vi "S_param_from_frame.VI"(2 "Ref Impedance":u16=75, 3 "S-parameter Array":cdb[][](array[numeric]) format="%.2f", 4 "Frequencies (Hz)":dbl[](array[numeric]) format="%.2e", 5 "Comments":string) -> (1 "Data Output":T1={"Comments"="", "Ref Impedance"=75, "Trace Array"=[]} {"Trace Array"."Freq (Hz)" format="%.2e"; "Trace Array"."S-parameter Array" format="%.2f"})   [LabVIEW 2017]
doc: "Writes data in Freq S Real Imag or Magnitude Angle \n9 Column Touchstone format \nfeatures write protection for existing files"
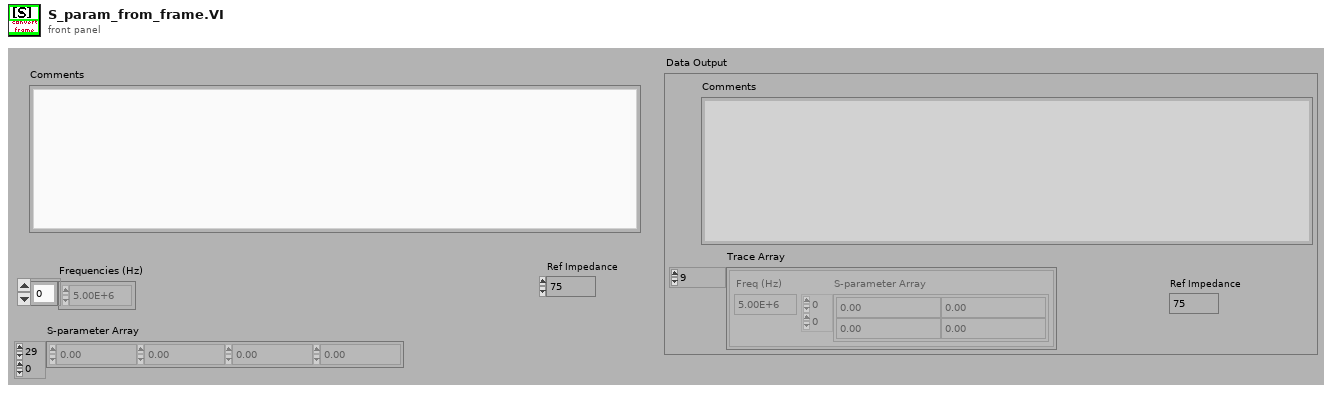
[diagram p1: front panel]
types:
  T1 = cluster{"Comments":string, "Ref Impedance":u16, "Trace Array":cluster{"Freq (Hz)":dbl, "S-parameter Array":cdb[][]}[]}
  T2 = cluster{"Freq (Hz)":dbl, "S-parameter Array":cdb[][]}[]
  T3 = cluster{"Freq (Hz)":dbl, "S-parameter Array":cdb[][]}
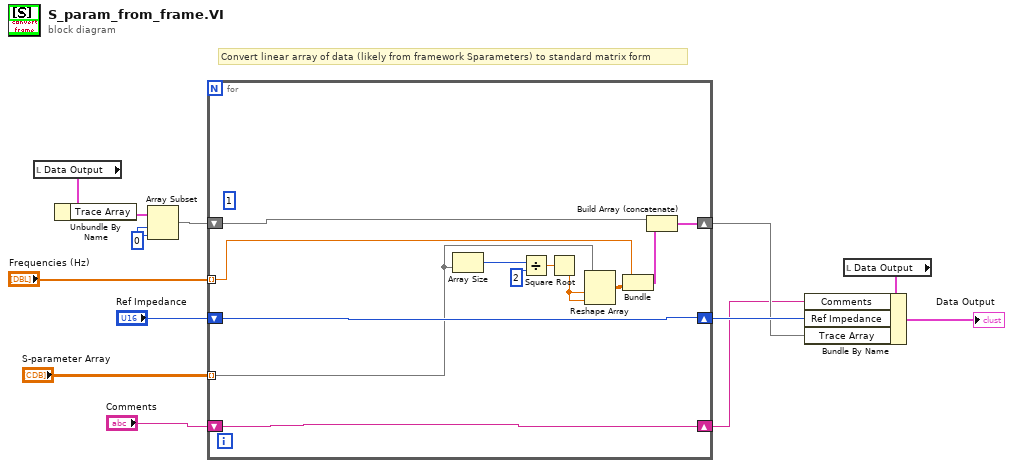
[diagram p0: block diagram]
diagram:
  w7 = 0
  # "Convert linear array of data (likely from framework Sparameters) to standard matrix form"
  n1 = local read "Data Output"() -> (w10:T1)
  n2 = Unbundle By Name(w10) -> ("Trace Array"=w9:T2)
  n3 = Array Subset(array=w9, index=w7, length=w7) -> (w8:T2)
  n4 = for {
    shift-right: [w25] -> w11
    shift-left: "Ref Impedance" -> [w25]
    shift-right: [w23] -> w6
    shift-left: w8 -> [w24]
    shift-right: [w22] -> w5
    shift-left: "Comments" -> [w22]
    tunnel: "Frequencies (Hz)" -> [w16] mode=indexing
    tunnel: "S-parameter Array" -> [w15] mode=indexing
    (unwired) 1
    n5 = Array Size(array=w15) -> (size(s)=w14:i32)
    n6 = Divide(x=w14, y=2) -> (x/y=w20:dbl)
    n7 = Square Root(x=w20) -> (sqrt(x)=w19:dbl)
    n8 = Reshape Array(w15, w19, w19) -> (w18:cdb[][])
    n9 = Bundle("Freq (Hz)"=w16, "S-parameter Array"=w18) -> (w17:T3)  [unwired: 1 out]
    n10 = Build Array (concatenate)(w24, w17) -> (w23:T2)
  }
  n11 = local read "Data Output"() -> (w12:T1)
  n12 = Bundle By Name(cluster=w12, "Comments"=w5, "Ref Impedance"=w11, "Trace Array"=w6) -> (→"Data Output":T1)
